vi "Configure Sweep Coupling Characteristics.vi"(0 "VISA resource name":refnum<visa-resource-name>, 1 "Auto FFT Width (T: Enable)":bool=TRUE, 2 "Manual FFT Width (0 Hz)":dbl, 5 "Sweep Type (0: Auto)":i32(ring) items=["Auto", "FFT", "Sweep"], 7 "Sweep Type Rules (0: Auto)":i32(ring) items=["Auto", "Best Speed", "Best Dynamic Range"], 9 "Sweep Time Rules (0: Auto)":i32(ring) items=["Auto", "Normal", "Accuracy", "Stimulus/Response"], 11 "error in (no error)":errorcluster, 12 "Auto SPAN/RBW Ratio (T: Enable)":bool=TRUE, 13 "Manual SPAN/RBW Ratio (106)":i32=106) -> (4 "VISA resource name out":refnum<visa-resource-name>, 15 "error out":errorcluster)   [LabVIEW 2018, in "Agilent MXA Series.lvlib"]
doc: "Configures the coupling and sweeping characteristics of the spectrum analyzer. \n\n<B>Note:</B>\nThis VI is applicable only when the measurement type is Swept SA, Channel Power, Occupied Bandwidth, ACP, Spurious Emissions or TOI."
uses:
  Agilent MXA Series.lvlib
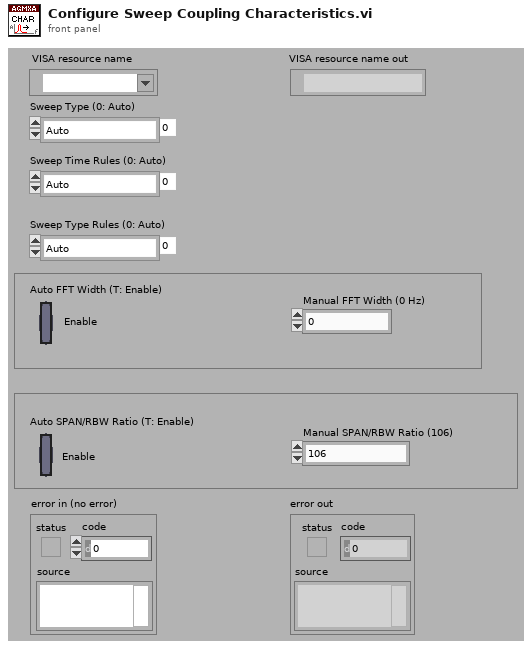
[diagram p1: front panel]
types:
  T1 = typedef "Agilent MXA Series.lvlib/Extended User Data.ctl" = cluster{"Measurement Type":i32, "Agilent MXA/EXA Model":i32}
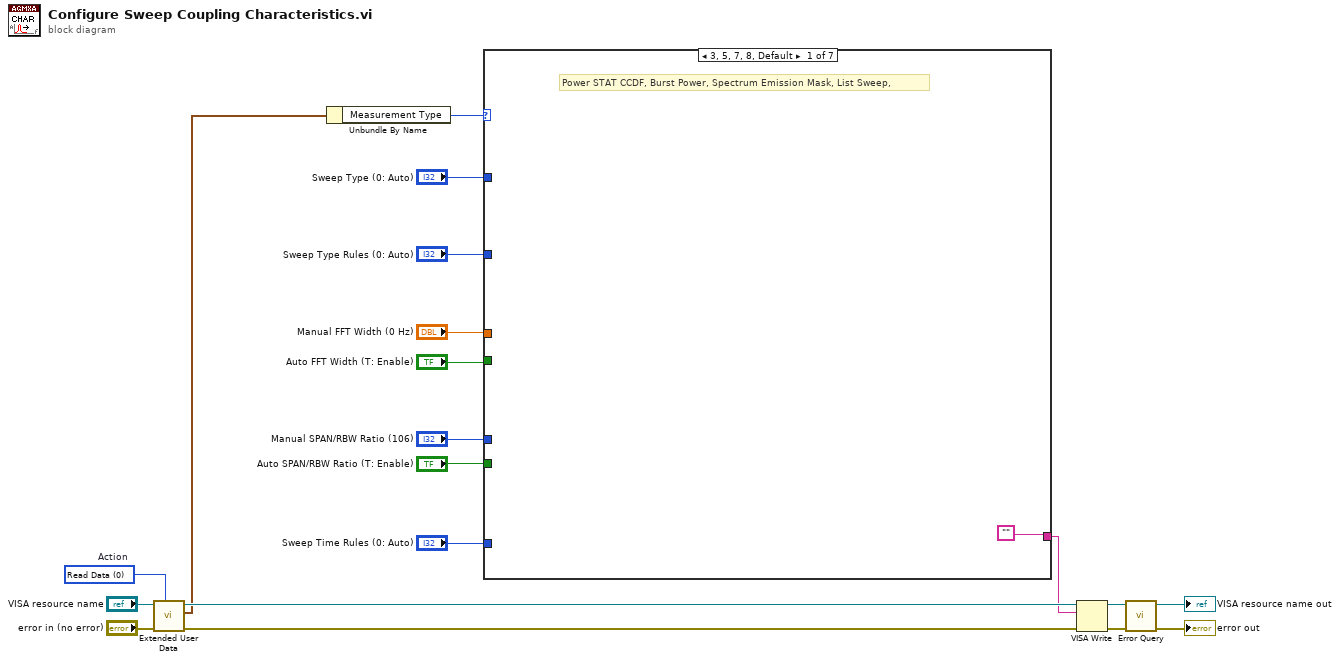
[diagram p0: block diagram]
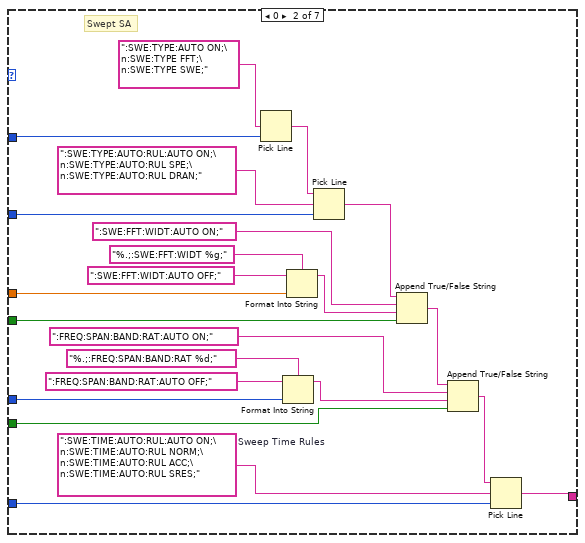
[diagram p2: hidden frame]
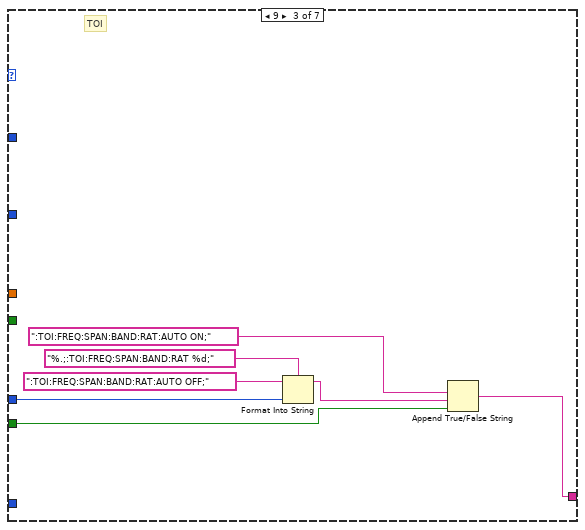
[diagram p3: hidden frame]
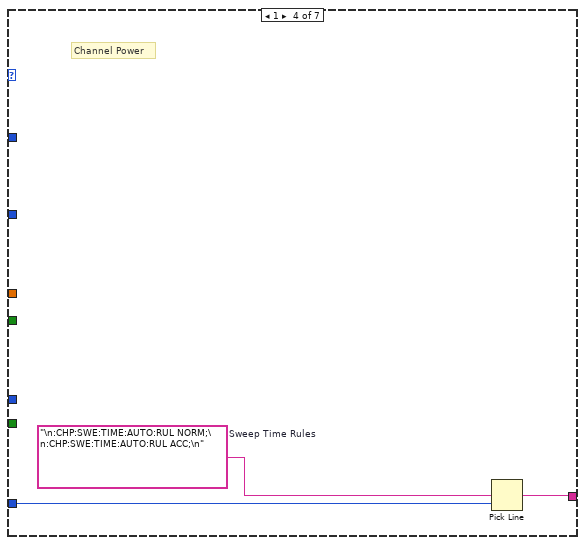
[diagram p4: hidden frame]
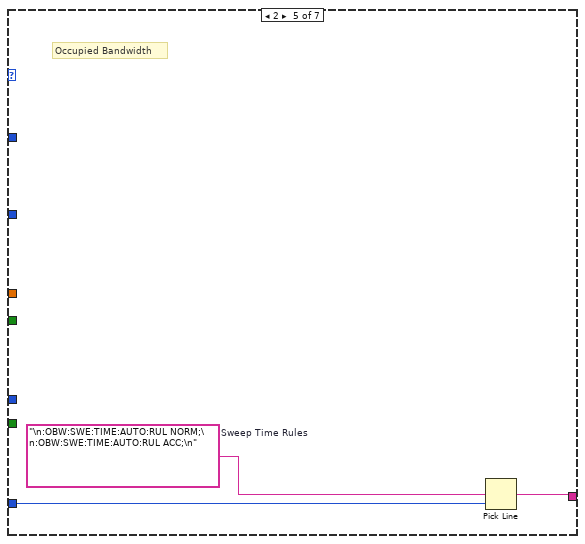
[diagram p5: hidden frame]
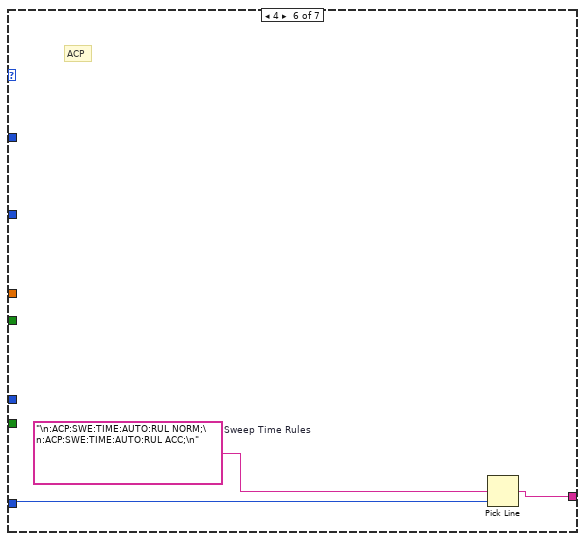
[diagram p6: hidden frame]
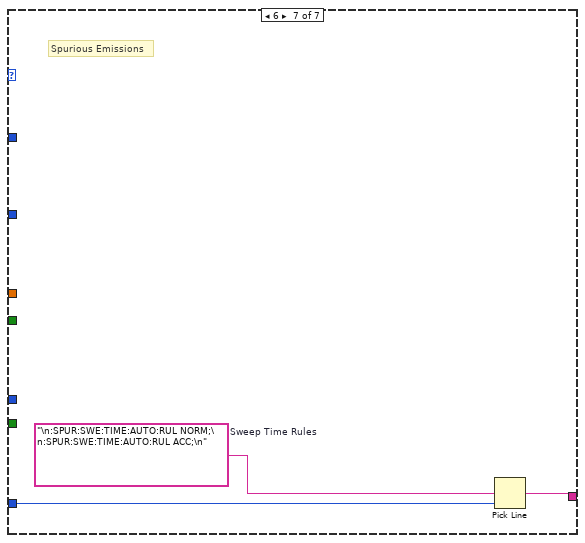
[diagram p7: hidden frame]
diagram:
  w13 = 0 items=["Read Data", "Write Data", "Clear Data", "Clear ALL Data"]  # Action
  n1 = call "Extended User Data.vi"("Action (1:Write Data)"=w13, "Error In (no error)"="error in (no error)", "VISA resource name in"="VISA resource name") -> ("Error Out"=w11:errorcluster, "User Data Out"=w10:T1, "VISA resource name out"=w12:refnum<visa-resource-name>)  [unwired: 6 in]
  n2 = Unbundle By Name(w10) -> ("Measurement Type"=w9:i32)
  n3 = case shown="3, 5, 7, 8, Default" w9 {
    tunnel: "Sweep Type (0: Auto)" -> [_ w35 _ _ _ _ _]
    tunnel: "Sweep Type Rules (0: Auto)" -> [_ w32 _ _ _ _ _]
    tunnel: "Manual FFT Width (0 Hz)" -> [_ w31 _ _ _ _ _]
    tunnel: "Auto FFT Width (T: Enable)" -> [_ w30 _ _ _ _ _]
    tunnel: "Manual SPAN/RBW Ratio (106)" -> [_ w29 w46 _ _ _ _]
    tunnel: "Auto SPAN/RBW Ratio (T: Enable)" -> [_ w28 w45 _ _ _ _]
    tunnel: "Sweep Time Rules (0: Auto)" -> [_ w26 _ w52 w55 w58 w60]
    tunnel: ["" ("output string") w21 w44 w51 w54 w57 w61] -> w1
    frame 3, 5, 7, 8, Default {
      # "Power STAT CCDF, Burst Power, Spectrum Emission Mask, List Sweep,"
    }
    frame 0 {
      w27 = ":SWE:TIME:AUTO:RUL:AUTO ON;\n:SWE:TIME:AUTO:RUL NORM;\n:SWE:TIME:AUTO:RUL ACC;\n:SWE:TIME:AUTO:RUL SRES;"  # Sweep Time Rules
      # "Swept SA"
      n4 = Pick Line(multi-line string=":SWE:TYPE:AUTO ON;\n:SWE:TYPE FFT;\n:SWE:TYPE SWE;", line index=w35) -> (output string=w25:string)  [unwired: 1 in]
      n5 = Format Into String(format string="%.;:FREQ:SPAN:BAND:RAT %d;", initial string=":FREQ:SPAN:BAND:RAT:AUTO OFF;" ("format string"), w29) -> (resulting string=w40:string)  [unwired: 1 in, 1 out]
      n6 = Format Into String(format string="%.;:SWE:FFT:WIDT %g;", initial string=":SWE:FFT:WIDT:AUTO OFF;" ("format string"), w31) -> (resulting string=w36:string)  [unwired: 1 in, 1 out]
      n7 = Pick Line(string ("")=w25, multi-line string=":SWE:TYPE:AUTO:RUL:AUTO ON;\n:SWE:TYPE:AUTO:RUL SPE;\n:SWE:TYPE:AUTO:RUL DRAN;", line index=w32) -> (output string=w24:string)
      n8 = Append True/False String(1:w30, 2:w36, 3:":SWE:FFT:WIDT:AUTO ON;" ("format string"), 4:w24) -> (0:w23:string)
      n9 = Append True/False String(1:w28, 2:w40, 3:":FREQ:SPAN:BAND:RAT:AUTO ON;" ("format string"), 4:w23) -> (0:w22:string)
      n10 = Pick Line(string ("")=w22, multi-line string=w27, line index=w26) -> (output string=w21:string)
    }
    frame 9 {
      # "TOI"
      n11 = Format Into String(format string="%.;:TOI:FREQ:SPAN:BAND:RAT %d;", initial string=":TOI:FREQ:SPAN:BAND:RAT:AUTO OFF;" ("format string"), w46) -> (resulting string=w47:string)  [unwired: 1 in, 1 out]
      n12 = Append True/False String(1:w45, 2:w47, 3:":TOI:FREQ:SPAN:BAND:RAT:AUTO ON;" ("format string")) -> (0:w44:string)  [unwired: 1 in]
    }
    frame 1 {
      w53 = "\n:CHP:SWE:TIME:AUTO:RUL NORM;\n:CHP:SWE:TIME:AUTO:RUL ACC;\n"  # Sweep Time Rules
      # "Channel Power"
      n13 = Pick Line(multi-line string=w53, line index=w52) -> (output string=w51:string)  [unwired: 1 in]
    }
    frame 2 {
      w56 = "\n:OBW:SWE:TIME:AUTO:RUL NORM;\n:OBW:SWE:TIME:AUTO:RUL ACC;\n"  # Sweep Time Rules
      # "Occupied Bandwidth"
      n14 = Pick Line(multi-line string=w56, line index=w55) -> (output string=w54:string)  [unwired: 1 in]
    }
    frame 4 {
      w59 = "\n:ACP:SWE:TIME:AUTO:RUL NORM;\n:ACP:SWE:TIME:AUTO:RUL ACC;\n"  # Sweep Time Rules
      # "ACP"
      n15 = Pick Line(multi-line string=w59, line index=w58) -> (output string=w57:string)  [unwired: 1 in]
    }
    frame 6 {
      w62 = "\n:SPUR:SWE:TIME:AUTO:RUL NORM;\n:SPUR:SWE:TIME:AUTO:RUL ACC;\n"  # Sweep Time Rules
      # "Spurious Emissions"
      n16 = Pick Line(multi-line string=w62, line index=w60) -> (output string=w61:string)  [unwired: 1 in]
    }
  }
  n17 = VISA Write(VISA resource name=w12, write buffer=w1, error in (no error)=w11) -> (VISA resource name out=w19:refnum<visa-resource-name>, error out=w17:errorcluster)  [unwired: 1 out]
  n18 = call "Error Query.vi"("error in (no error)"=w17, "VISA resource name"=w19) -> ("error out"=→"error out":errorcluster, "VISA resource name out"=→"VISA resource name out":refnum<visa-resource-name>)  [unwired: 6 in, 2 out]
